vi "LEP_RV_LinkerFlags.vi"(1 "Build configuration":u16(ring) items=["Debug", "Release"]) -> (0 "LFlags":string)   [LabVIEW 2011]
doc: "Returns the linker flags for a given embedded target and <B>Build configuration</B>."
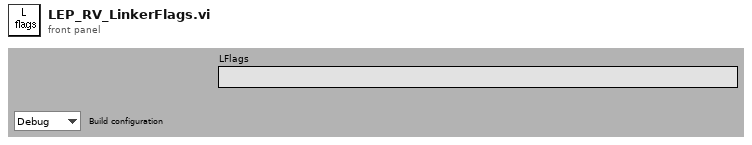
[diagram p1: front panel]
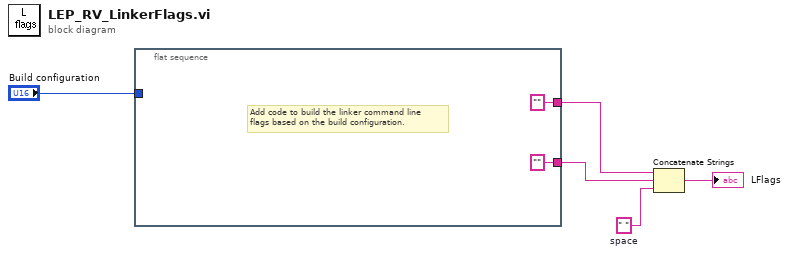
[diagram p0: block diagram]
diagram:
  w1 = " "  # space
  n1 = flat-sequence {
    tunnel: [""] -> w5
    tunnel: "Build configuration" -> [_]
    tunnel: [""] -> w2
    frame #0 {
      # "Add code to build the linker command line\nflags based on the build configuration."
    }
  }
  n2 = Concatenate Strings(w2, w5, w1) -> (→"LFlags":string)
